vi "MW_DeviceType.vi"() -> (2 "DeviceType":T1)   [LabVIEW 2016, in "Microwave Source.lvlib"]
uses:
  Microwave Source.lvlib
  MW_ctl_DeviceType.ctl
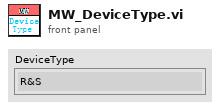
[diagram p1: front panel]
types:
  T1 = typedef "Microwave Source.lvlib/MW_ctl_DeviceType.ctl" = enum16{"R&S", "Other"}
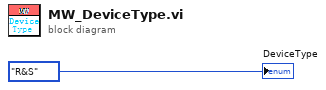
[diagram p0: block diagram]
diagram:
  "DeviceType" <- MW_ctl_DeviceType."R&S" ("DeviceType")
